vi "create_sample_calibration_rois.vi"() -> ()   [LabVIEW 2019]
uses:
  <vilib>/vision/Image Controls.llb/IMAQ Image.ctl
panel:
  in  "ROI Size":i32
  in  "Number of ROIs":i32
  out "Image Out":T1
  in  "Image":T1
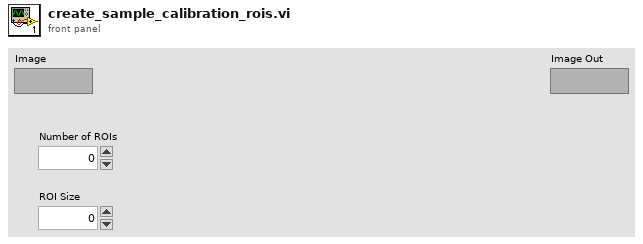
[diagram p1: front panel]
types:
  T1 = typedef "IMAQ Image.ctl" = refnum<image>
  T2 = typedef "ROI Descriptor" = cluster{"Global Rectangle":i32[], "Contours":cluster{"ID":enum32{"External", "Internal"}, "Type":u32, "Coordinates":i32[]}[]}
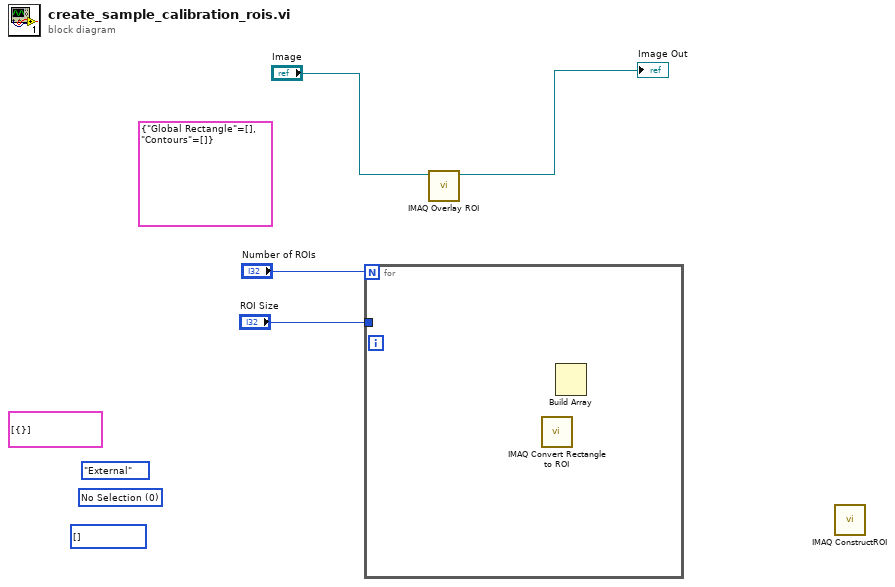
[diagram p0: block diagram]
diagram:
  (unwired) i32[] [] ("Coordinates")
  (unwired) u32 0 items=["No Selection", "Point", "Line", "Rectangle", "Oval", "Polygon", "Freehand Region", "Annulus", "Unused2", "Unused3", "Broken Line", "Freehand Line", "Rotated Rectangle"] ("Type")
  (unwired) enum32{"External", "Internal"}."External" ("ID")
  (unwired) cluster{}[] [{}] ("Contours")
  (unwired) T2 {"Global Rectangle"=[], "Contours"=[]} ("ROI Descriptor")
  n1 = for {
    N: "Number of ROIs" -> [_]
    tunnel: "ROI Size" -> [_]
    n2 = call "IMAQ Convert Rectangle to ROI"() -> ()  [unwired: 9 in, 2 out]
    n3 = Build Array() -> ()  [unwired: 4 in, 1 out]
  }
  n4 = call "IMAQ Overlay ROI"("Image"="Image") -> ("Image Out"=→"Image Out":T1)  [unwired: 9 in, 1 out]
  n5 = call "IMAQ ConstructROI"() -> ()  [unwired: 8 in, 4 out]
